vi "WPI_DriverStationStart Communication.vi"(8 "error in (no error)":errorcluster, 11 "occurrence":refnum<k4>) -> ()   [LabVIEW 2017]
doc: "Starts the communication loop between the CompactRIO device and the driver station. This VI also initializes the host computer, joystick, and driver station data caches, as well as the system watchdog on the CompactRIO device.\n\nThis software is licensed. Open the labview\\readme\\WPI Robotics Library Open Source License.txt file for more information."
uses:
  <vilib>/Rock Robotics/SystemInterfaces/NetworkCommunication/NetComm_UsageReport_ResourceType.ctl
panel:
  # "This VI start the communication loop and cache data for LabVIEW."
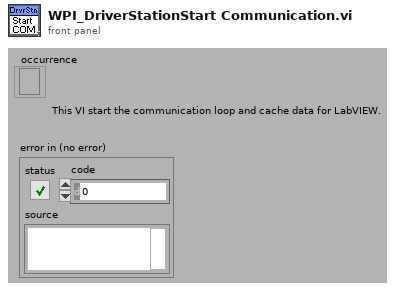
[diagram p1: front panel]
types:
  T1 = typedef "NetComm_UsageReport_ResourceType.ctl" = enum8{"Controller", "Module", "Language", "CANPlugin", "Accelerometer", "ADXL345", "AnalogChannel", "AnalogTrigger", "AnalogTriggerOutput", "CANJaguar", "Compressor", "Counter", "Dashboard", "DigitalInput", "DigitalOutput", "DriverStationCIO", "DriverStationEIO", "DriverStationLCD", "Encoder", "GearTooth", "Gyro", "I2C", "Framework", "Jaguar", "Joystick", "Kinect", "KinectStick", "PIDController", "Preferences", "PWM", "Relay", "RobotDrive", "SerialPort", "Servo", "Solenoid", "SPI", "Task", "Ultrasonic", "Victor", "Button", "Command", "AxisCamera", "PCVideoServer", "SmartDashboard", "Talon", "HiTechnicColorSensor", "HiTechnicAccel", "HiTechnicCompass", "SRF08", "AnalogOutput", "Victor SP", "Talon SRX", "CAN Talon SRX", "ADXL362 Accel", "ADXRS450 Gyro", "Rev SPARK", "Mindsensors SD540", "Digital Filter", "ADIS16448", "PDP", "PCM", "PigeonIMU", "Nidec Brushless", "CTRE CANifier", "CTRE Future 0", "CTRE Future 1", "CTRE Future 2", "CTRE Future 3", "CTRE Future 4", "CTRE Future 5", "CTRE Future 6"}
  T2 = typedef "NetComm_ControlWord.ctl" = cluster{"Enabled":bool, "Autonomous":bool, "Test":bool, "E-Stop":bool, "FMS Attached":bool, "DS Attached":bool}
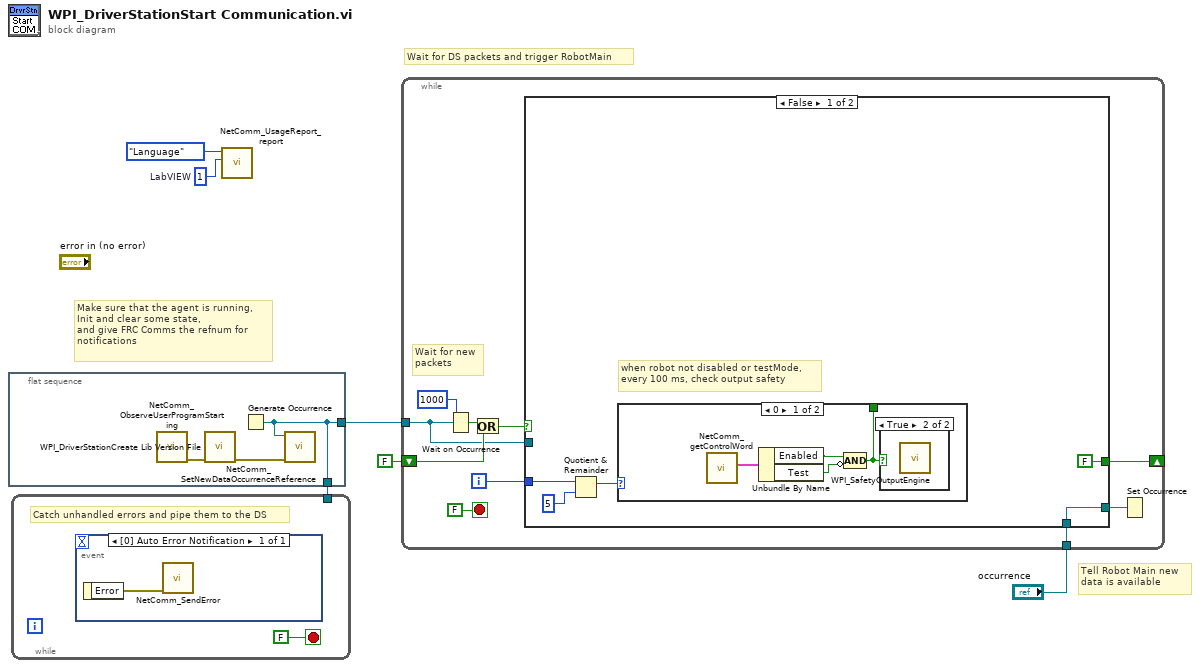
[diagram p0: block diagram]
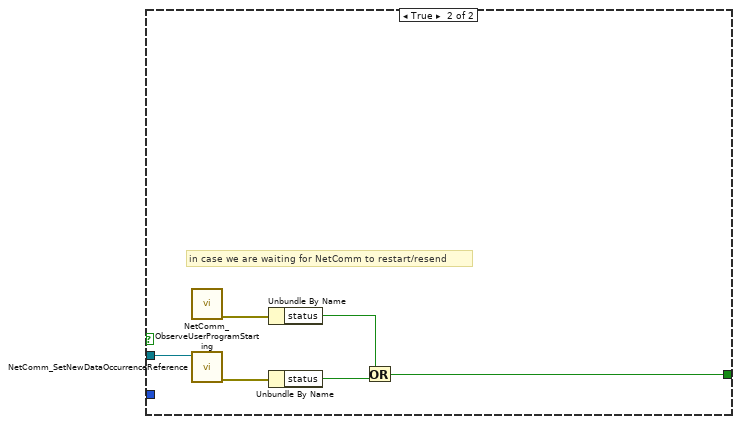
[diagram p4: hidden frame]
diagram:
  w3 = u8 1  # LabVIEW
  # "Tell Robot Main new\ndata is available"
  # "Wait for DS packets and trigger RobotMain"
  # "Make sure that the agent is running,\nInit and clear some state,\nand give FRC Comms the refnum for\nnotifications"
  n1 = flat-sequence {
    tunnel: [w7] -> w6
    tunnel: [w7] -> w2
    frame #0 {
      n2 = call <vilib>:"NetComm_ObserveUserProgramStarting.vi"() -> ("error out"=w8:errorcluster)  [unwired: 11 in]
      n3 = call <vilib>:"WPI_DriverStationCreate Lib Version File.vi"("error in"=w8) -> ("error out"=w9:errorcluster)  [unwired: 10 in]
      n4 = Generate Occurrence() -> (w7:refnum<k4>)
      n5 = call <vilib>:"NetComm_SetNewDataOccurrenceReference.vi"("error in"=w9, "occurrence"=w7) -> ()  [unwired: 10 out]
    }
  }
  n6 = while {
    tunnel: w2 -> [_]
    stop <- FALSE stop-if-true
    # "Catch unhandled errors and pipe them to the DS"
    n7 = event shown="[0] Auto Error Notification" {
      selector: _ -> [_]
      dyn-events: _ -> [_]
      timeout: _ -> [_]
      event Auto Error Notification {
        n8 = event-data() -> ("Error"=w11:errorcluster)  [unwired: 1 in]
        n9 = call <vilib>:"NetComm_SendError.vi"("error in (no error)"=w11) -> ()  [unwired: 11 in]
      }
    }
  }
  n10 = call <vilib>:"NetComm_UsageReport_report.vi"("Instance Number"=w3, "Resource Type"=NetComm_UsageReport_ResourceType."Language") -> ()  [unwired: 10 in]
  n11 = while {
    tunnel: w6 -> [w12]
    tunnel: "occurrence" -> [w17]
    shift-right: [w14] -> _
    shift-left: FALSE -> [w13]
    i -> [w19]
    stop <- FALSE stop-if-true
    # "Wait for new\npackets"
    n12 = Wait on Occurrence(2:w12, 3:1000 ("ms timeout (-1)")) -> (0:w20:bool)  [unwired: 1 out]
    n13 = Or(x=w20, y=w13) -> (x .or. y?=w15:bool)
    n14 = case shown="False" w15 {
      tunnel: w19 -> [w24 _]
      tunnel: w17 -> [w23 _]
      tunnel: [w23 _] -> w16
      tunnel: [FALSE w33] -> w14
      tunnel: w12 -> [_ w31]
      frame False {
        # "when robot not disabled or testMode,\nevery 100 ms, check output safety"
        n15 = Quotient & Remainder(x=w24, y=u32 5 ("milliseconds to wait")) -> (x-y*floor(x/y)=w25:u32)  [unwired: 1 out]
        n16 = case shown="0" w25 {
          tunnel: [w30 _] -> _
          frame 0 {
            n17 = call <vilib>:"NetComm_getControlWord.vi"() -> ("Control Word"=w29:T2)  [unwired: 10 in, 1 out]
            n18 = Unbundle By Name(w29) -> ("Enabled"=w28:bool, "Test"=w27:bool)
            n19 = Compound Arithmetic op=AND(w28, invert w27) -> (w30:bool)
            n20 = case shown="True" w30 {
              frame False {
              }
              frame True {
                n21 = call <vilib>:"WPI_SafetyOutputEngine.vi"() -> ()  [unwired: 1 out]
              }
            }
          }
          frame Default {
          }
        }
      }
      frame True {
        # "in case we are waiting for NetComm to restart/resend"
        n22 = call <vilib>:"NetComm_ObserveUserProgramStarting.vi"() -> ("error out"=w36:errorcluster)  [unwired: 11 in]
        n23 = call <vilib>:"NetComm_SetNewDataOccurrenceReference.vi"("occurrence"=w31) -> ("error out"=w35:errorcluster)  [unwired: 1 in, 9 out]
        n24 = Unbundle By Name(w36) -> ("status"=w32:bool)
        n25 = Unbundle By Name(w35) -> ("status"=w34:bool)
        n26 = Or(x=w32, y=w34) -> (x .or. y?=w33:bool)
      }
    }
    n27 = Set Occurrence(w16) -> ()
  }
